vi "公式写入.vi"(7 "公式":cluster{"X^2":dbl, "X":dbl, "b":dbl}, 8 "Error in":errorcluster caption="Error in (no error)", 9 "量程选择":enum16{"低量程1", "低量程2", "高量程1", "高量程2"}(ring), 10 "测量模式(公式)":u16(ring)=1 items=["水样测试"=1, "标样核查"=2, "零点核查"=3, "跨度核查"=4, "空白测试"=5, "平行样"=6, "加标回收"=7], 11 "模型":enum32{"线性", "多项式"}(ring)) -> (0 "error out":errorcluster)   [LabVIEW 2016, in "斯坦道CODMn.lvlib"]
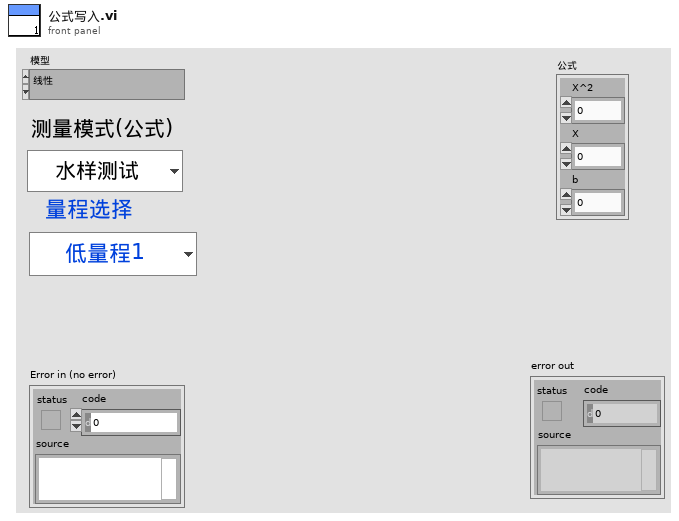
[diagram p1: front panel]
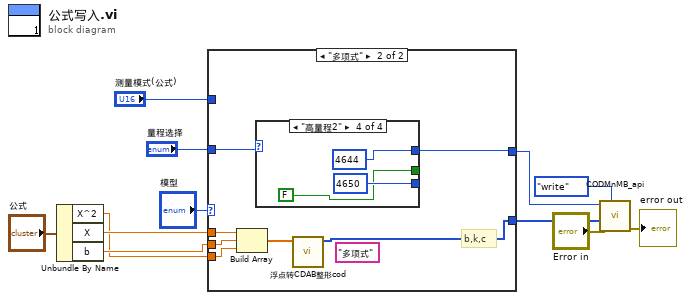
[diagram p0: block diagram]
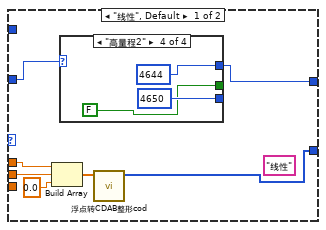
[diagram p2: hidden frame]
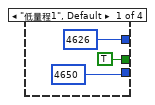
[diagram p3: hidden frame]
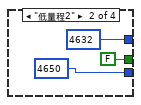
[diagram p4: hidden frame]
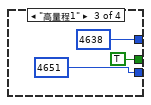
[diagram p5: hidden frame]
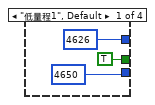
[diagram p6: hidden frame]
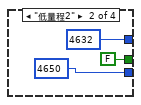
[diagram p7: hidden frame]
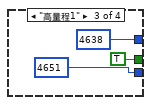
[diagram p8: hidden frame]
diagram:
  n1 = Unbundle By Name("公式") -> ("X^2"=w6:dbl, "X"=w7:dbl, "b"=w8:dbl)
  n2 = case shown="\"多项式\"" "模型" {
    tunnel: [w14 w32] -> w5
    tunnel: [w18 w37] -> w9
    tunnel: w8 -> [w16 w34]
    tunnel: w7 -> [w17 w35]
    tunnel: w6 -> [_ w36]
    tunnel: "测量模式(公式)" -> [_ _]
    tunnel: "量程选择" -> [w13 w33]
    frame "线性", Default {
      (unwired) "线性" ("table输入")
      n3 = Build Array(w17, w16, 0.0 ("元素")) -> (w19:dbl[])
      n4 = case shown="\"高量程2\"" w13 {
        tunnel: [u16 4626 ("starting address") u16 4632 ("starting address") u16 4638 ("starting address") u16 4644 ("starting address")] -> w14
        tunnel: [u16 4650 ("starting address") u16 4650 ("starting address") u16 4651 ("starting address") u16 4650 ("starting address")] -> _
        tunnel: [TRUE FALSE TRUE FALSE] -> _
        frame "低量程1", Default {
        }
        frame "低量程2" {
        }
        frame "高量程1" {
        }
        frame "高量程2" {
        }
      }
      n5 = call "浮点转CDAB整形cod.vi"("浮点数"=w19) -> ("CDAB整形输出"=w18:u16[])  [unwired: 10 in]
    }
    frame "多项式" {
      (unwired) "多项式" ("table输入")
      # "b,k,c"
      n6 = Build Array(w35, w34, w36) -> (w38:dbl[])
      n7 = case shown="\"高量程2\"" w33 {
        tunnel: [u16 4626 ("starting address") u16 4632 ("starting address") u16 4638 ("starting address") u16 4644 ("starting address")] -> w32
        tunnel: [u16 4650 ("starting address") u16 4650 ("starting address") u16 4651 ("starting address") u16 4650 ("starting address")] -> _
        tunnel: [TRUE FALSE TRUE FALSE] -> _
        frame "低量程1", Default {
        }
        frame "低量程2" {
        }
        frame "高量程1" {
        }
        frame "高量程2" {
        }
      }
      n8 = call "浮点转CDAB整形cod.vi"("浮点数"=w38) -> ("CDAB整形输出"=w37:u16[])  [unwired: 10 in]
    }
  }
  n9 = call "CODMnMB_api.vi"("STEP"=enum16{"open", "read", "write", "close"}."write", "Error in"="Error in", "values"=w9, "starting address"=w5) -> ("error out"=→"error out":errorcluster)  [unwired: 5 in, 2 out]
